vi "HB_SendHeader.vi"(8 "error in (no error)":errorcluster, 10 "Header":string, 11 "SerialPortRef":T1) -> (0 "error out":errorcluster, 3 "SerialPortRef 2":T1)   [LabVIEW 2016]
uses:
  <vilib>/Rock Robotics/WPI/SerialPort/WPI_SerialPortRef.ctl
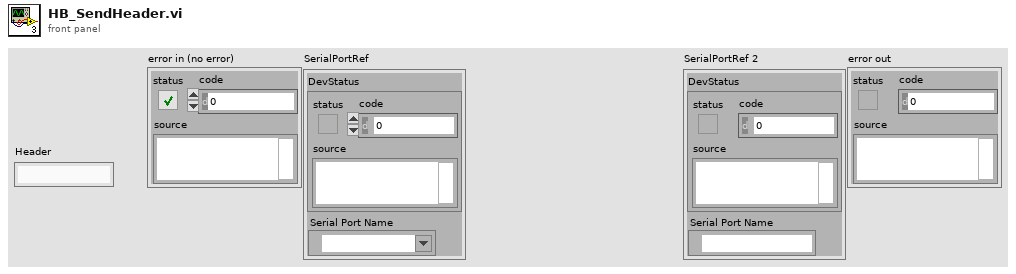
[diagram p1: front panel]
types:
  T1 = typedef "WPI_SerialPortRef.ctl" = cluster{"DevStatus":errorcluster, "Serial Port Name":refnum<visa-resource-name>}
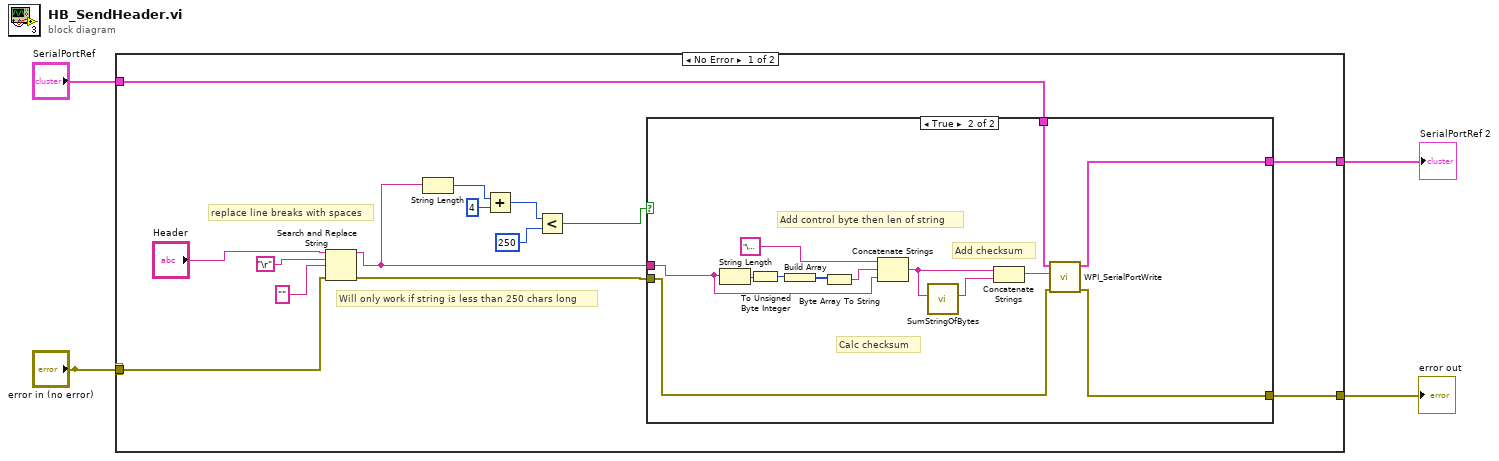
[diagram p0: block diagram]
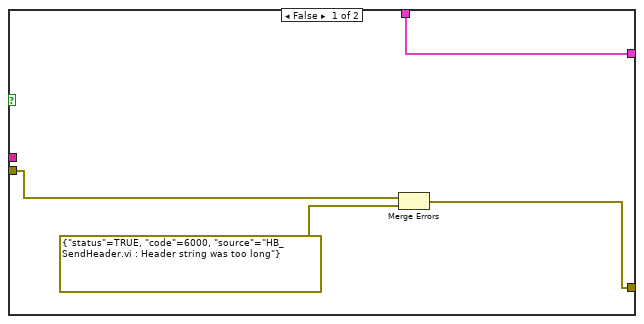
[diagram p2: hidden frame]
diagram:
  n1 = case shown="No Error" "error in (no error)" {
    selector: "error in (no error)" -> [_ w36]
    tunnel: "error in (no error)" -> [w11 _]
    tunnel: "SerialPortRef" -> [w7 w37]
    tunnel: [w6 w36] -> w3
    tunnel: [w5 w37] -> w2
    frame No Error {
      # "Will only work if string is less than 250 chars long"
      # "replace line breaks with spaces"
      n2 = Search and Replace String(input string="Header", search string="\r", replace string="" ("replace string (\"\")"), error in=w11) -> (result string=w8:string, error out=w12:errorcluster)  [unwired: 4 in, 2 out]
      n3 = String Length(string=w8) -> (length=w10:i32)
      n4 = Add(x=w10, y=4) -> (x+y=w14:i32)
      n5 = Less?(x=w14, y=250) -> (x < y?=w9:bool)
      n6 = case shown="True" w9 {
        tunnel: w12 -> [w22 w27]
        tunnel: w8 -> [_ w26]
        tunnel: w7 -> [w19 w25]
        tunnel: [w20 w24] -> w6
        tunnel: [w19 w23] -> w5
        frame False {
          n7 = Merge Errors(w22, errorcluster {"status"=TRUE, "code"=6000, "source"="HB_SendHeader.vi : Header string was too long"} ("error out")) -> (w20:errorcluster)
        }
        frame True {
          # "Calc checksum"
          # "Add checksum"
          # "Add control byte then len of string"
          n8 = String Length(string=w26) -> (length=w34:i32)
          n9 = To Unsigned Byte Integer(number=w34) -> (unsigned 8bit integer=w31:u8)
          n10 = Build Array(w31) -> (w32:u8[])
          n11 = Byte Array To String(unsigned byte array=w32) -> (string=w33:string)
          n12 = Concatenate Strings("\u0002", w33, w26) -> (w29:string)
          n13 = call "SumStringOfBytes.vi"("String Of Bytes"=w29) -> ("SumAsString"=w28:string)  [unwired: 10 in]
          n14 = Concatenate Strings(w29, w28) -> (w35:string)
          n15 = call <vilib>:"WPI_SerialPortWrite.vi"("error in (no error)"=w27, "Buffer"=w35, "SerialPortRef"=w25) -> ("error out"=w24:errorcluster, "SerialPortRef"=w23:T1)  [unwired: 6 in, 1 out]
        }
      }
    }
    frame Error {
    }
  }
  "SerialPortRef 2" <- w2
  "error out" <- w3
